vi "register status change event.vi"(11 "generate status number":i32=100) -> (3 "status number":i32)   [LabVIEW 2017, in "testcase-Basic-Function.lvclass"]
uses:
  testcase-Basic-Function.lvclass
  f9bca660-bddd-4266-99d8-d96952150cc2.vi
  src/user.lib/_NEVSTOP/Communicable State Machine(CSM)/Communicable State Machine.lvlib
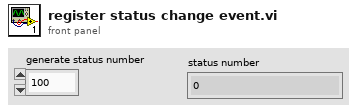
[diagram p1: front panel]
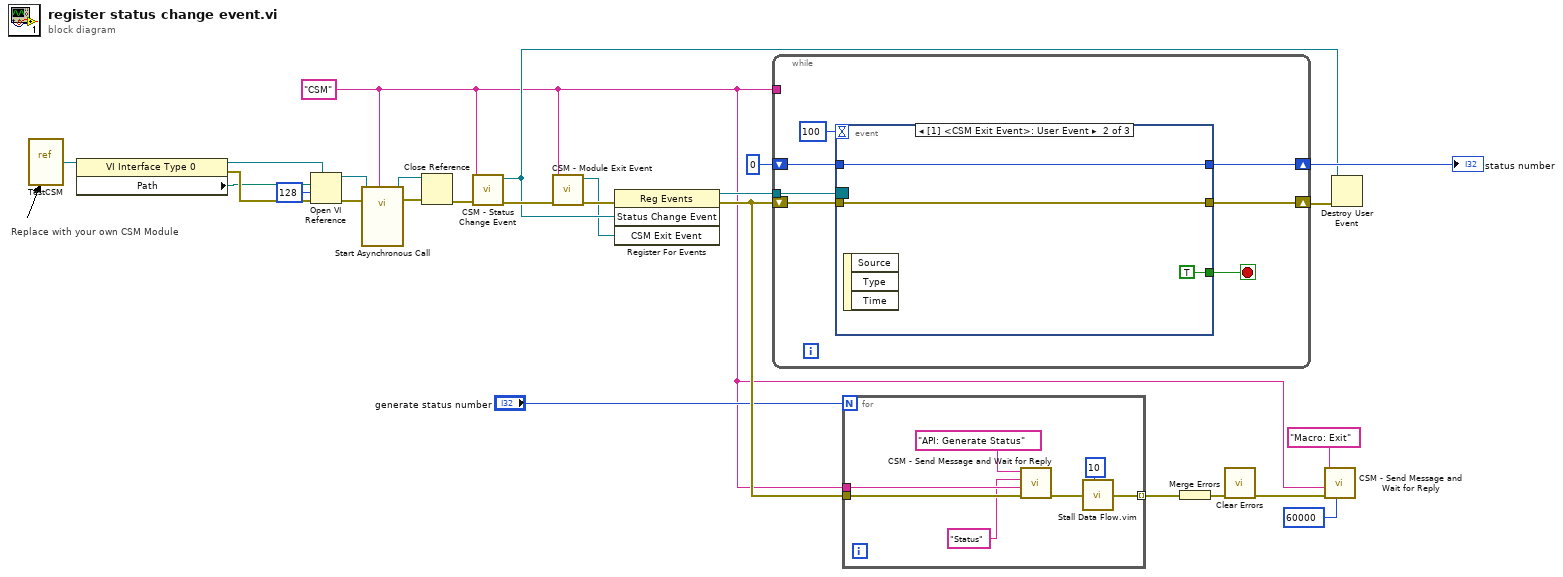
[diagram p0: block diagram]
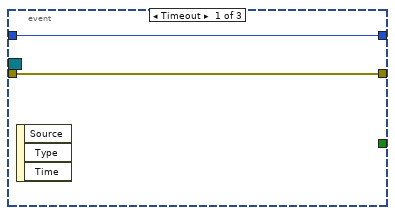
[diagram p2: hidden frame]
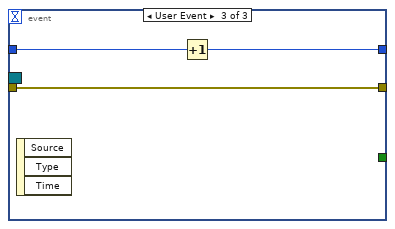
[diagram p3: hidden frame]
diagram:
  w4 = "CSM" ("Name (\"\" to Use UUID)")
  # "Replace with your own CSM Module"
  n1 = vi-ref "TestCSM.vi"() -> (w19:refnum<vi>)
  n2 = property class="VI Interface Type 0"(reference=w19) -> (reference out=w23:refnum<vi>, error out=w21:errorcluster, "Path"=w20:path)  [unwired: 1 in]
  n3 = Open VI Reference(type specifier VI Refnum (for type only)=w23, vi path=w20, options=128, error in (no error)=w21) -> (vi reference=w22:refnum<vi>, error out=w18:errorcluster)  [unwired: 2 in]
  n4 = call-by-ref "Start Asynchronous Call"(reference=w22, error in=w18, "Name(\"\" to use uuid)"=w4) -> (reference out=w25:refnum<vi>, error out=w24:errorcluster)  [unwired: 11 in]
  n5 = Close Reference(reference=w25, error in (no error)=w24) -> (error out=w17:errorcluster)
  n6 = call "CSM - Status Change Event.vi"("Error In"=w17, "CSM Module"=w4) -> ("error out"=w16:errorcluster, "Status Change Event"=w6:refnum<user-event>)  [unwired: 7 in, 1 out]
  n7 = call "CSM - Module Exit Event.vi"("Error In"=w16, "Name (\"\" to Use UUID) In"=w4) -> ("error out"=w5:errorcluster, "CSM Exit Event"=w3:refnum<user-event>)  [unwired: 7 in, 1 out]
  n8 = register-events(error in=w5, w6, w3) -> (reference out=w15:refnum<event-registration>, error out=w14:errorcluster)  [unwired: 1 in]
  n9 = while {
    tunnel: w15 -> [w33]
    tunnel: w4 -> [_]
    shift-right: [w29] -> w8
    shift-left: 0 -> [w31]
    shift-right: [w28] -> w7
    shift-left: w14 -> [w32]
    stop <- w27 stop-if-true
    n10 = event shown="[1] <CSM Exit Event>: User Event" {
      selector: w33 -> [_ _ _]
      dyn-events: _ -> [_ _ _]
      timeout: 100 -> [_ _ _]
      tunnel: w32 -> [w34 w37 w39]
      tunnel: w31 -> [w35 w38 w41]
      tunnel: [w35 w38 w40] -> w29
      tunnel: [w34 w37 w39] -> w28
      tunnel: [_ TRUE _] -> w27
      event Timeout {
        n11 = event-data() -> ()  [unwired: 1 in, 3 out]
      }
      event User Event {
        n12 = event-data() -> ()  [unwired: 1 in, 3 out]
      }
      event User Event {
        n13 = event-data() -> ()  [unwired: 1 in, 3 out]
        n14 = Increment(x=w41) -> (x+1=w40:i32)
      }
    }
  }
  "status number" <- w8
  n15 = for {
    N: "generate status number" -> [_]
    tunnel: w14 -> [w48]
    tunnel: w4 -> [w47]
    tunnel: [w43] -> w12 mode=indexing
    n16 = call "CSM - Send Message and Wait for Reply.vi"("Error In (No Error)"=w48, "Target Module"=w47, "Arguments (\"\")"="Status" ("Arguments (\"\")"), "State"="API: Generate Status") -> ("error out"=w44:errorcluster)  [unwired: 5 in, 2 out]
    n17 = call "Stall Data Flow.vim"("value in"=w44, "milliseconds to wait"=10) -> ("value out"=w43:errorcluster)  [unwired: 1 out]
  }
  n18 = Merge Errors(w12) -> (w11:errorcluster)
  n19 = call <vilib>:"Clear Errors.vi"("error in (no error)"=w11) -> ("error out"=w2:errorcluster)  [unwired: 5 in, 1 out]
  n20 = call "CSM - Send Message and Wait for Reply.vi"("Response Timeout (-2 Using Global Settings)"=60000, "Error In (No Error)"=w2, "Target Module"=w4, "State"="Macro: Exit") -> ()  [unwired: 5 in, 3 out]
  n21 = Destroy User Event(user event=w6, error in=w7) -> ()  [unwired: 1 out]
